vi "Version_4.9_8_on-chip_valves_for25ulSyringe_withModfied_Plunging.vi"() -> ()   [LabVIEW 2020] (continued)
                                tunnel: [w4564 w4571] -> w4555
                                tunnel: w4557 -> [w4563 w4572]
                                frame "Standard Pumping", Default {
                                n4147 = Subtract(x=w4565, y=w4566) -> (x-y=w4562:dbl)
                                n4148 = Absolute Value(x=w4562) -> (abs(x)=w4561:dbl)
                                n4149 = Multiply(x=w4561, y=w4563) -> (x*y=w4568:dbl)
                                n4150 = Divide(x=w4568, y=3000.0) -> (x/y=w4564:dbl)
                                }
                                frame "High Resolution Pumping" {
                                n4151 = Subtract(x=w4574, y=w4573) -> (x-y=w4570:dbl)
                                n4152 = Absolute Value(x=w4570) -> (abs(x)=w4569:dbl)
                                n4153 = Multiply(x=w4569, y=w4572) -> (x*y=w4576:dbl)
                                n4154 = Divide(x=w4576, y=24000.0) -> (x/y=w4571:dbl)
                                }
                                }
                                n4155 = local write "Volume being Injected \nin this process"(w4555) -> ()
                                }
                                frame #1 {
                                n4156 = call "LSPOneStatus (SubVI).vi"("VISA Refnum in"=w4580) -> ("read buffer"=w4582:string)  [unwired: 10 in]
                                n4157 = call <vilib>:"Trim Whitespace.vi"("string"=w4582) -> ("trimmed string"=w4581:string)  [unwired: 1 in]
                                n4158 = local read "Stopper that ends \nthe main loops"() -> (w4577:bool)
                                n4159 = Equal?(x=w4581, y="/0`\u0003") -> (x = y?=w4579:bool)
                                n4160 = Or(x=w4579, y=w4577) -> (x .or. y?=w4578:bool)
                                }
                                }
                                n4161 = Wait (ms)(milliseconds to wait=u32 100) -> ()  [unwired: 1 out]
                                n4162 = local read "Stopper that ends \nthe main loops"() -> (w4547:bool)
                                n4163 = case shown="True" w4547 {
                                frame False {
                                }
                                frame True {
                                n4164 = local read "VISA Refnum in\nfor Pump"() -> (w4554:refnum<visa-resource-name>)
                                n4165 = call "HardStopCurrentProcess (SubVI).vi"("VISA Refnum in"=w4554) -> ()  [unwired: 11 in]
                                }
                                }
                                }
                              }
                              frame #7 {
                                # "Change the pump port to Buffer-A1 for equilibriation of column-1"
                                n4166 = local read "VISA Refnum in\nfor Pump"() -> (w4585:refnum<visa-resource-name>)
                                n4167 = local read "Port for \nA1-Equilibriation"() -> (w4584:string)
                                n4168 = local write "Pause Data Collection"(TRUE ("Pause Data Collection")) -> ()
                                n4169 = Wait (ms)(milliseconds to wait=u32 500) -> ()  [unwired: 1 out]
                                n4170 = call "PortChanger (SubVI).vi"("Port Number"=w4584, "VISA Refnum in"=w4585) -> ()  [unwired: 10 in]
                              }
                              frame #8 {
                                n4171 = local read "VISA Refnum in\nfor Pump"() -> (w4589:refnum<visa-resource-name>)
                                n4172 = local write "Volume being Injected \nin this process"(0.0 ("Volume being Injected \nin this process")) -> ()
                                n4173 = call "ProcessCompletionWaiter (SubVI).vi"("VISA Refnum in"=w4589) -> ()  [unwired: 11 in]
                                n4174 = local write "Start the Process"(FALSE ("Start the Process")) -> ()
                              }
                            }
                          }
                          frame #7 {
                            # "Clean the tubing with Buffer-A1"
                            n4175 = local read "N-A1"() -> (w4591:i32)
                            n4176 = for {
                              N: w4591 -> [_]
                              n4177 = stacked-sequence {
                                frame #0 {
                                n4178 = local read "VISA Refnum in\nfor Pump"() -> (w4594:refnum<visa-resource-name>)
                                n4179 = local read "Port for \nA1-Equilibriation"() -> (w4593:string)
                                n4180 = call "PortChanger (SubVI).vi"("Port Number"=w4593, "VISA Refnum in"=w4594) -> ()  [unwired: 10 in]
                                }
                                frame #1 {
                                n4181 = local read "VISA Refnum in\nfor Pump"() -> (w4595:refnum<visa-resource-name>)
                                n4182 = call "ProcessCompletionWaiter (SubVI).vi"("VISA Refnum in"=w4595) -> ()  [unwired: 11 in]
                                }
                                frame #2 {
                                n4183 = local read "VISA Refnum in\nfor Pump"() -> (w4600:refnum<visa-resource-name>)
                                n4184 = local read "Apparent Volume\nof Syringe"() -> (w4596:dbl)
                                n4185 = local read "Volume of Syringe"() -> (w4597:dbl)
                                n4186 = call "RPickUp(SubVI).vi"("Volume to be picked up"=w4596, "Volume of Syringe"=w4597, "Resolution of PickUP"=T2."Standard Pumping", "PickUp Flow Rate (ul/min)"=150.0, "VISA Refnum in"=w4600) -> ()  [unwired: 6 in, 1 out]
                                }
                                frame #3 {
                                n4187 = local read "Stopper that ends \nthe main loops"() -> (w4601:bool)
                                n4188 = local read "VISA Refnum in\nfor Pump"() -> (w4602:refnum<visa-resource-name>)
                                n4189 = case shown="True" w4601 {
                                frame False {
                                }
                                frame True {
                                n4190 = local read "VISA Refnum in\nfor Pump"() -> (w4603:refnum<visa-resource-name>)
                                n4191 = call "HardStopCurrentProcess (SubVI).vi"("VISA Refnum in"=w4603) -> ()  [unwired: 11 in]
                                }
                                }
                                n4192 = call "ProcessCompletionWaiter (SubVI).vi"("VISA Refnum in"=w4602) -> ()  [unwired: 11 in]
                                }
                                frame #4 {
                                n4193 = local read "VISA Refnum in\nfor Pump"() -> (w4605:refnum<visa-resource-name>)
                                n4194 = call "PortChanger (SubVI).vi"("Port Number"="1", "VISA Refnum in"=w4605) -> ()  [unwired: 10 in]
                                }
                                frame #5 {
                                n4195 = local read "Stopper that ends \nthe main loops"() -> (w4606:bool)
                                n4196 = local read "VISA Refnum in\nfor Pump"() -> (w4607:refnum<visa-resource-name>)
                                n4197 = case shown="True" w4606 {
                                frame False {
                                }
                                frame True {
                                n4198 = local read "VISA Refnum in\nfor Pump"() -> (w4608:refnum<visa-resource-name>)
                                n4199 = call "HardStopCurrentProcess (SubVI).vi"("VISA Refnum in"=w4608) -> ()  [unwired: 11 in]
                                }
                                }
                                n4200 = call "ProcessCompletionWaiter (SubVI).vi"("VISA Refnum in"=w4607) -> ()  [unwired: 11 in]
                                }
                                frame #6 {
                                n4201 = local read "VISA Refnum in\nfor Pump"() -> (w4613:refnum<visa-resource-name>)
                                n4202 = local read "Volume of Syringe"() -> (w4610:dbl)
                                n4203 = call "GoToAbsolutePosition(SubVI).vi"("Absolute Volume Position in Syringe (in ul)"=0.0 ("Volume to be picked up"), "Volume of Syringe"=w4610, "Resolution of Pumping"=T2."Standard Pumping" ("Resolution of PickUP"), "Flow Rate (ul/min)"=150.0 ("PickUp Flow Rate (ul/min)"), "VISA Refnum in"=w4613) -> ()  [unwired: 6 in, 1 out]
                                }
                                frame #7 {
                                n4204 = local read "Stopper that ends \nthe main loops"() -> (w4614:bool)
                                n4205 = local read "VISA Refnum in\nfor Pump"() -> (w4615:refnum<visa-resource-name>)
                                n4206 = case shown="True" w4614 {
                                frame False {
                                }
                                frame True {
                                n4207 = local read "VISA Refnum in\nfor Pump"() -> (w4616:refnum<visa-resource-name>)
                                n4208 = call "HardStopCurrentProcess (SubVI).vi"("VISA Refnum in"=w4616) -> ()  [unwired: 11 in]
                                }
                                }
                                n4209 = call "ProcessCompletionWaiter (SubVI).vi"("VISA Refnum in"=w4615) -> ()  [unwired: 11 in]
                                }
                              }
                              n4210 = local write "Pause Data Collection"(TRUE ("Pause Data Collection")) -> ()
                            }
                          }
                          frame #8 {
                            # "Switch to Port-4"
                            # "Port-4 of pump is connected to Buffer-A1"
                            n4211 = local read "Port for \nA1-Equilibriation"() -> (w4617:string)
                            n4212 = local read "VISA Refnum in\nfor Pump"() -> (w4618:refnum<visa-resource-name>)
                            n4213 = call "PortChanger (SubVI).vi"("Port Number"=w4617, "VISA Refnum in"=w4618) -> ()  [unwired: 10 in]
                          }
                          frame #9 {
                            n4214 = local read "VISA Refnum in\nfor Pump"() -> (w4619:refnum<visa-resource-name>)
                            n4215 = call "ProcessCompletionWaiter (SubVI).vi"("VISA Refnum in"=w4619) -> ()  [unwired: 11 in]
                          }
                          frame #10 {
                            # "External vale is temporarily connected to teh waste outlet in this code"
                            n4216 = local write "Valve V3 Open"(FALSE ("Valve V3 Open")) -> ()
                            n4217 = local write "Valve V4 Open"(FALSE ("Valve V4 Open")) -> ()
                            n4218 = local write "Valve V1 Open"(TRUE ("Valve V1 Open")) -> ()
                            n4219 = local write "Valve V2 Open"(TRUE ("Valve V2 Open")) -> ()
                            n4220 = local write "External Valve \nOpen"(TRUE ("External Valve \nOpen")) -> ()
                            n4221 = local write "Valve V8 Open"(FALSE ("Valve V8 Open")) -> ()
                            n4222 = local write "Valve V6 Open"(FALSE ("Valve V6 Open")) -> ()
                            n4223 = local write "Valve V5 Open"(FALSE ("Valve V5 Open")) -> ()
                            n4224 = local write "Valve V7 Open"(FALSE ("Valve V7 Open")) -> ()
                          }
                          frame #11 {
                            n4225 = local read "Buffer-A1 Volume \nto be  Pumped \nfor Equilibration\nof Column-1"() -> (w4632:dbl)
                            n4226 = local read "Apparent Volume\nof Syringe"() -> (w4629:dbl)
                            n4227 = Quotient & Remainder(x=w4632, y=w4629) -> (x-y*floor(x/y)=w4630:dbl, floor(x/y)=w4631:dbl)
                            n4228 = for {
                              N: w4631 -> [_]
                              n4229 = stacked-sequence {
                                frame #0 {
                                n4230 = local read "Buffer-A1 PickUp \nFlow Rate (ul/min)\nfor Equilibration \nof Column-1"() -> (w4635:dbl)
                                n4231 = local read "Buffer-A1 Pumping\nResolution \nfor Equilibration \nof Column-1"() -> (w4634:T2)
                                n4232 = local read "VISA Refnum in\nfor Pump"() -> (w4637:refnum<visa-resource-name>)
                                n4233 = local read "Apparent Volume\nof Syringe"() -> (w4633:dbl)
                                n4234 = local read "Volume of Syringe"() -> (w4636:dbl)
                                n4235 = call "RPickUp(SubVI).vi"("Volume to be picked up"=w4633, "Volume of Syringe"=w4636, "Resolution of PickUP"=w4634, "PickUp Flow Rate (ul/min)"=w4635, "VISA Refnum in"=w4637) -> ()  [unwired: 6 in, 1 out]
                                }
                                frame #1 {
                                n4236 = while {
                                stop <- w4638 stop-if-true
                                n4237 = local read "Stopper that ends \nthe main loops"() -> (w4639:bool)
                                n4238 = local read "VISA Refnum in\nfor Pump"() -> (w4640:refnum<visa-resource-name>)
                                n4239 = case shown="True" w4639 {
                                frame False {
                                }
                                frame True {
                                n4240 = local read "VISA Refnum in\nfor Pump"() -> (w4641:refnum<visa-resource-name>)
                                n4241 = call "HardStopCurrentProcess (SubVI).vi"("VISA Refnum in"=w4641) -> ()  [unwired: 11 in]
                                }
                                }
                                n4242 = call "ProcessCompletionWaiterWithOutPut (SubVI).vi"("VISA Refnum in"=w4640) -> ("Boolean"=w4638:bool)  [unwired: 10 in]
                                }
                                }
                                frame #2 {
                                # "Reads the initial Plunger Position for computing the volume dispensed"
                                n4243 = local read "VISA Refnum in\nfor Pump"() -> (w4643:refnum<visa-resource-name>)
                                n4244 = call "AbsolutePlungerPosition (SubVI).vi"("VISA Refnum in"=w4643) -> ("Plunger Position"=w4642:i32)  [unwired: 10 in]
                                n4245 = local write "Initial Plunger Position"(w4642) -> ()
                                }
                                frame #3 {
                                # "Switch to Port-2"
                                # "Port-2 of the pump is conncted to column-1 of chip"
                                n4246 = local read "VISA Refnum in\nfor Pump"() -> (w4645:refnum<visa-resource-name>)
                                n4247 = call "PortChanger (SubVI).vi"("Port Number"="2", "VISA Refnum in"=w4645) -> ()  [unwired: 10 in]
                                }
                                frame #4 {
                                n4248 = while {
                                stop <- w4646 stop-if-true
                                n4249 = local read "Stopper that ends \nthe main loops"() -> (w4647:bool)
                                n4250 = local read "VISA Refnum in\nfor Pump"() -> (w4648:refnum<visa-resource-name>)
                                n4251 = case shown="True" w4647 {
                                frame False {
                                }
                                frame True {
                                n4252 = local read "VISA Refnum in\nfor Pump"() -> (w4649:refnum<visa-resource-name>)
                                n4253 = call "HardStopCurrentProcess (SubVI).vi"("VISA Refnum in"=w4649) -> ()  [unwired: 11 in]
                                }
                                }
                                n4254 = call "ProcessCompletionWaiterWithOutPut (SubVI).vi"("VISA Refnum in"=w4648) -> ("Boolean"=w4646:bool)  [unwired: 10 in]
                                }
                                }
                                frame #5 {
                                n4255 = local read "Buffer-A1 Dispense\nFlow Rate (ul/min) \nfor Equilibration\nof Column-1"() -> (w4653:dbl)
                                n4256 = local read "Buffer-A1 Pumping\nResolution \nfor Equilibration \nof Column-1"() -> (w4652:T2)
                                n4257 = local read "VISA Refnum in\nfor Pump"() -> (w4655:refnum<visa-resource-name>)
                                n4258 = local write "Pause Data Collection"(FALSE ("Pause Data Collection")) -> ()
                                n4259 = local read "Volume of Syringe"() -> (w4654:dbl)
                                n4260 = call "GoToAbsolutePosition(SubVI).vi"("Absolute Volume Position in Syringe (in ul)"=0.0, "Volume of Syringe"=w4654, "Resolution of Pumping"=w4652, "Flow Rate (ul/min)"=w4653, "VISA Refnum in"=w4655) -> ()  [unwired: 6 in, 1 out]
                                }
                                frame #6 {
                                n4261 = local read "Buffer-A1 Pumping\nResolution \nfor Equilibration \nof Column-1"() -> (w4657:T2)
                                n4262 = local read "VISA Refnum in\nfor Pump"() -> (w4659:refnum<visa-resource-name>)
                                n4263 = local read "Initial Plunger Position"() -> (w4658:dbl)
                                n4264 = local read "Volume of Syringe"() -> (w4656:dbl)
                                n4265 = while {
                                tunnel: w4658 -> [w4666]
                                tunnel: w4659 -> [w4665]
                                tunnel: w4657 -> [w4664]
                                tunnel: w4656 -> [w4663]
                                stop <- w4661 stop-if-true
                                n4266 = stacked-sequence {
                                tunnel: w4666 -> [w4673 _]
                                tunnel: w4665 -> [w4672 w4693]
                                tunnel: w4664 -> [w4671 _]
                                tunnel: w4663 -> [w4670 _]
                                tunnel: [_ w4691] -> w4661
                                frame #0 {
                                n4267 = call "AbsolutePlungerPosition (SubVI).vi"("VISA Refnum in"=w4672) -> ("Plunger Position"=w4669:i32)  [unwired: 10 in]
                                n4268 = case shown="\"Standard Pumping\", Default" w4671 {
                                tunnel: w4673 -> [w4678 w4687]
                                tunnel: w4669 -> [w4679 w4686]
                                tunnel: [w4677 w4684] -> w4668
                                tunnel: w4670 -> [w4676 w4685]
                                frame "Standard Pumping", Default {
                                n4269 = Subtract(x=w4678, y=w4679) -> (x-y=w4675:dbl)
                                n4270 = Absolute Value(x=w4675) -> (abs(x)=w4674:dbl)
                                n4271 = Multiply(x=w4674, y=w4676) -> (x*y=w4681:dbl)
                                n4272 = Divide(x=w4681, y=3000.0) -> (x/y=w4677:dbl)
                                }
                                frame "High Resolution Pumping" {
                                n4273 = Subtract(x=w4687, y=w4686) -> (x-y=w4683:dbl)
                                n4274 = Absolute Value(x=w4683) -> (abs(x)=w4682:dbl)
                                n4275 = Multiply(x=w4682, y=w4685) -> (x*y=w4689:dbl)
                                n4276 = Divide(x=w4689, y=24000.0) -> (x/y=w4684:dbl)
                                }
                                }
                                n4277 = local write "Volume being Injected \nin this process"(w4668) -> ()
                                }
                                frame #1 {
                                n4278 = call "LSPOneStatus (SubVI).vi"("VISA Refnum in"=w4693) -> ("read buffer"=w4695:string)  [unwired: 10 in]
                                n4279 = call <vilib>:"Trim Whitespace.vi"("string"=w4695) -> ("trimmed string"=w4694:string)  [unwired: 1 in]
                                n4280 = local read "Stopper that ends \nthe main loops"() -> (w4690:bool)
                                n4281 = Equal?(x=w4694, y="/0`\u0003") -> (x = y?=w4692:bool)
                                n4282 = Or(x=w4692, y=w4690) -> (x .or. y?=w4691:bool)
                                }
                                }
                                n4283 = Wait (ms)(milliseconds to wait=u32 100) -> ()  [unwired: 1 out]
                                n4284 = local read "Stopper that ends \nthe main loops"() -> (w4660:bool)
                                n4285 = case shown="True" w4660 {
                                frame False {
                                }
                                frame True {
                                n4286 = local read "VISA Refnum in\nfor Pump"() -> (w4667:refnum<visa-resource-name>)
                                n4287 = call "HardStopCurrentProcess (SubVI).vi"("VISA Refnum in"=w4667) -> ()  [unwired: 11 in]
                                }
                                }
                                }
                                }
                                frame #7 {
                                # "Change the pump port back to Buffer-A1"
                                n4288 = local read "VISA Refnum in\nfor Pump"() -> (w4698:refnum<visa-resource-name>)
                                n4289 = local read "Port for \nA1-Equilibriation"() -> (w4697:string)
                                n4290 = local write "Pause Data Collection"(TRUE ("Pause Data Collection")) -> ()
                                n4291 = Wait (ms)(milliseconds to wait=u32 500) -> ()  [unwired: 1 out]
                                n4292 = call "PortChanger (SubVI).vi"("Port Number"=w4697, "VISA Refnum in"=w4698) -> ()  [unwired: 10 in]
                                }
                                frame #8 {
                                n4293 = local read "VISA Refnum in\nfor Pump"() -> (w4701:refnum<visa-resource-name>)
                                n4294 = local write "Volume being Injected \nin this process"(0.0 ("Volume being Injected \nin this process")) -> ()
                                n4295 = call "ProcessCompletionWaiter (SubVI).vi"("VISA Refnum in"=w4701) -> ()  [unwired: 11 in]
                                }
                              }
                            }
                            n4296 = local write "Reminder of the \nVolume to be \nPumped"(w4630) -> ()
                          }
                          frame #12 {
                            n4297 = stacked-sequence {
                              frame #0 {
                                n4298 = local read "Buffer-A1 PickUp \nFlow Rate (ul/min)\nfor Equilibration \nof Column-1"() -> (w4705:dbl)
                                n4299 = local read "Buffer-A1 Pumping\nResolution \nfor Equilibration \nof Column-1"() -> (w4704:T2)
                                n4300 = local read "VISA Refnum in\nfor Pump"() -> (w4707:refnum<visa-resource-name>)
                                n4301 = local read "Reminder of the \nVolume to be \nPumped"() -> (w4703:dbl)
                                n4302 = local read "Volume of Syringe"() -> (w4706:dbl)
                                n4303 = call "RPickUp(SubVI).vi"("Volume to be picked up"=w4703, "Volume of Syringe"=w4706, "Resolution of PickUP"=w4704, "PickUp Flow Rate (ul/min)"=w4705, "VISA Refnum in"=w4707) -> ()  [unwired: 6 in, 1 out]
                              }
                              frame #1 {
                                n4304 = while {
                                stop <- w4708 stop-if-true
                                n4305 = local read "Stopper that ends \nthe main loops"() -> (w4709:bool)
                                n4306 = local read "VISA Refnum in\nfor Pump"() -> (w4710:refnum<visa-resource-name>)
                                n4307 = case shown="True" w4709 {
                                frame False {
                                }
                                frame True {
                                n4308 = local read "VISA Refnum in\nfor Pump"() -> (w4711:refnum<visa-resource-name>)
                                n4309 = call "HardStopCurrentProcess (SubVI).vi"("VISA Refnum in"=w4711) -> ()  [unwired: 11 in]
                                }
                                }
                                n4310 = call "ProcessCompletionWaiterWithOutPut (SubVI).vi"("VISA Refnum in"=w4710) -> ("Boolean"=w4708:bool)  [unwired: 10 in]
                                }
                              }
                              frame #2 {
                                # "Reads the initial Plunger Position for computing the volume dispensed"
                                n4311 = local read "VISA Refnum in\nfor Pump"() -> (w4713:refnum<visa-resource-name>)
                                n4312 = call "AbsolutePlungerPosition (SubVI).vi"("VISA Refnum in"=w4713) -> ("Plunger Position"=w4712:i32)  [unwired: 10 in]
                                n4313 = local write "Initial Plunger Position"(w4712) -> ()
                              }
                              frame #3 {
                                # "Switch to Port-2"
                                # "Port-2 of the pump is conncted to column-1 of chip"
                                n4314 = local read "VISA Refnum in\nfor Pump"() -> (w4715:refnum<visa-resource-name>)
                                n4315 = call "PortChanger (SubVI).vi"("Port Number"="2", "VISA Refnum in"=w4715) -> ()  [unwired: 10 in]
                              }
                              frame #4 {
                                n4316 = while {
                                stop <- w4716 stop-if-true
                                n4317 = local read "Stopper that ends \nthe main loops"() -> (w4717:bool)
                                n4318 = local read "VISA Refnum in\nfor Pump"() -> (w4718:refnum<visa-resource-name>)
                                n4319 = case shown="True" w4717 {
                                frame False {
                                }
                                frame True {
                                n4320 = local read "VISA Refnum in\nfor Pump"() -> (w4719:refnum<visa-resource-name>)
                                n4321 = call "HardStopCurrentProcess (SubVI).vi"("VISA Refnum in"=w4719) -> ()  [unwired: 11 in]
                                }
                                }
                                n4322 = call "ProcessCompletionWaiterWithOutPut (SubVI).vi"("VISA Refnum in"=w4718) -> ("Boolean"=w4716:bool)  [unwired: 10 in]
                                }
                              }
                              frame #5 {
                                n4323 = local read "Buffer-A1 Pumping\nResolution \nfor Equilibration \nof Column-1"() -> (w4722:T2)
                                n4324 = local read "Buffer-A1 Dispense\nFlow Rate (ul/min) \nfor Equilibration\nof Column-1"() -> (w4723:dbl)
                                n4325 = local read "VISA Refnum in\nfor Pump"() -> (w4725:refnum<visa-resource-name>)
                                n4326 = local write "Pause Data Collection"(FALSE ("Pause Data Collection")) -> ()
                                n4327 = local read "Volume of Syringe"() -> (w4724:dbl)
                                n4328 = call "GoToAbsolutePosition(SubVI).vi"("Absolute Volume Position in Syringe (in ul)"=0.0 ("Volume to be Dispensed"), "Volume of Syringe"=w4724, "Resolution of Pumping"=w4722, "Flow Rate (ul/min)"=w4723, "VISA Refnum in"=w4725) -> ()  [unwired: 6 in, 1 out]
                              }
                              frame #6 {
                                n4329 = local read "Buffer-A1 Pumping\nResolution \nfor Equilibration \nof Column-1"() -> (w4727:T2)
                                n4330 = local read "VISA Refnum in\nfor Pump"() -> (w4729:refnum<visa-resource-name>)
                                n4331 = local read "Initial Plunger Position"() -> (w4728:dbl)
                                n4332 = local read "Volume of Syringe"() -> (w4726:dbl)
                                n4333 = while {
                                tunnel: w4728 -> [w4736]
                                tunnel: w4729 -> [w4735]
                                tunnel: w4727 -> [w4734]
                                tunnel: w4726 -> [w4733]
                                stop <- w4731 stop-if-true
                                n4334 = stacked-sequence {
                                tunnel: w4736 -> [w4743 _]
                                tunnel: w4735 -> [w4742 w4763]
                                tunnel: w4734 -> [w4741 _]
                                tunnel: w4733 -> [w4740 _]
                                tunnel: [_ w4761] -> w4731
                                frame #0 {
                                n4335 = call "AbsolutePlungerPosition (SubVI).vi"("VISA Refnum in"=w4742) -> ("Plunger Position"=w4739:i32)  [unwired: 10 in]
                                n4336 = case shown="\"Standard Pumping\", Default" w4741 {
                                tunnel: w4743 -> [w4748 w4757]
                                tunnel: w4739 -> [w4749 w4756]
                                tunnel: [w4747 w4754] -> w4738
                                tunnel: w4740 -> [w4746 w4755]
                                frame "Standard Pumping", Default {
                                n4337 = Subtract(x=w4748, y=w4749) -> (x-y=w4745:dbl)
                                n4338 = Absolute Value(x=w4745) -> (abs(x)=w4744:dbl)
                                n4339 = Multiply(x=w4744, y=w4746) -> (x*y=w4751:dbl)
                                n4340 = Divide(x=w4751, y=3000.0) -> (x/y=w4747:dbl)
                                }
                                frame "High Resolution Pumping" {
                                n4341 = Subtract(x=w4757, y=w4756) -> (x-y=w4753:dbl)
                                n4342 = Absolute Value(x=w4753) -> (abs(x)=w4752:dbl)
                                n4343 = Multiply(x=w4752, y=w4755) -> (x*y=w4759:dbl)
                                n4344 = Divide(x=w4759, y=24000.0) -> (x/y=w4754:dbl)
                                }
                                }
                                n4345 = local write "Volume being Injected \nin this process"(w4738) -> ()
                                }
                                frame #1 {
                                n4346 = call "LSPOneStatus (SubVI).vi"("VISA Refnum in"=w4763) -> ("read buffer"=w4765:string)  [unwired: 10 in]
                                n4347 = call <vilib>:"Trim Whitespace.vi"("string"=w4765) -> ("trimmed string"=w4764:string)  [unwired: 1 in]
                                n4348 = local read "Stopper that ends \nthe main loops"() -> (w4760:bool)
                                n4349 = Equal?(x=w4764, y="/0`\u0003") -> (x = y?=w4762:bool)
                                n4350 = Or(x=w4762, y=w4760) -> (x .or. y?=w4761:bool)
                                }
                                }
                                n4351 = Wait (ms)(milliseconds to wait=u32 100) -> ()  [unwired: 1 out]
                                n4352 = local read "Stopper that ends \nthe main loops"() -> (w4730:bool)
                                n4353 = case shown="True" w4730 {
                                frame False {
                                }
                                frame True {
                                n4354 = local read "VISA Refnum in\nfor Pump"() -> (w4737:refnum<visa-resource-name>)
                                n4355 = call "HardStopCurrentProcess (SubVI).vi"("VISA Refnum in"=w4737) -> ()  [unwired: 11 in]
                                }
                                }
                                }
                              }
                              frame #7 {
                                # "Change the pump port to Buffer-C1 for equilibriation of column-2"
                                n4356 = local read "VISA Refnum in\nfor Pump"() -> (w4768:refnum<visa-resource-name>)
                                n4357 = local read "Port for \nC1-Equilibriation"() -> (w4767:string)
                                n4358 = local write "Pause Data Collection"(TRUE ("Pause Data Collection")) -> ()
                                n4359 = Wait (ms)(milliseconds to wait=u32 500) -> ()  [unwired: 1 out]
                                n4360 = call "PortChanger (SubVI).vi"("Port Number"=w4767, "VISA Refnum in"=w4768) -> ()  [unwired: 10 in]
                              }
                              frame #8 {
                                n4361 = local read "VISA Refnum in\nfor Pump"() -> (w4772:refnum<visa-resource-name>)
                                n4362 = local write "Volume being Injected \nin this process"(0.0 ("Volume being Injected \nin this process")) -> ()
                                n4363 = call "ProcessCompletionWaiter (SubVI).vi"("VISA Refnum in"=w4772) -> ()  [unwired: 11 in]
                                n4364 = local write "Start the Process"(FALSE ("Start the Process")) -> ()
                              }
                            }
                          }
                          frame #13 {
                            # "Clean the tubing with Buffer-C1"
                            n4365 = local read "N-C1"() -> (w4775:i32)
                            n4366 = local write "Equilibriating \nColumn-1"(FALSE ("Equilibriating \nColumn-1")) -> ()
                            n4367 = for {
                              N: w4775 -> [_]
                              n4368 = stacked-sequence {
                                frame #0 {
                                n4369 = local read "Port for \nC1-Equilibriation"() -> (w4778:string)
                                n4370 = local read "VISA Refnum in\nfor Pump"() -> (w4779:refnum<visa-resource-name>)
                                n4371 = call "PortChanger (SubVI).vi"("Port Number"=w4778, "VISA Refnum in"=w4779) -> ()  [unwired: 10 in]
                                }
                                frame #1 {
                                n4372 = local read "VISA Refnum in\nfor Pump"() -> (w4780:refnum<visa-resource-name>)
                                n4373 = call "ProcessCompletionWaiter (SubVI).vi"("VISA Refnum in"=w4780) -> ()  [unwired: 11 in]
                                }
                                frame #2 {
                                n4374 = local read "VISA Refnum in\nfor Pump"() -> (w4785:refnum<visa-resource-name>)
                                n4375 = local read "Apparent Volume\nof Syringe"() -> (w4781:dbl)
                                n4376 = local read "Volume of Syringe"() -> (w4782:dbl)
                                n4377 = call "RPickUp(SubVI).vi"("Volume to be picked up"=w4781, "Volume of Syringe"=w4782, "Resolution of PickUP"=T2."Standard Pumping", "PickUp Flow Rate (ul/min)"=150.0, "VISA Refnum in"=w4785) -> ()  [unwired: 6 in, 1 out]
                                }
                                frame #3 {
                                n4378 = local read "Stopper that ends \nthe main loops"() -> (w4786:bool)
                                n4379 = local read "VISA Refnum in\nfor Pump"() -> (w4787:refnum<visa-resource-name>)
                                n4380 = case shown="True" w4786 {
                                frame False {
                                }
                                frame True {
                                n4381 = local read "VISA Refnum in\nfor Pump"() -> (w4788:refnum<visa-resource-name>)
                                n4382 = call "HardStopCurrentProcess (SubVI).vi"("VISA Refnum in"=w4788) -> ()  [unwired: 11 in]
                                }
                                }
                                n4383 = call "ProcessCompletionWaiter (SubVI).vi"("VISA Refnum in"=w4787) -> ()  [unwired: 11 in]
                                }
                                frame #4 {
                                n4384 = local read "VISA Refnum in\nfor Pump"() -> (w4790:refnum<visa-resource-name>)
                                n4385 = call "PortChanger (SubVI).vi"("Port Number"="1", "VISA Refnum in"=w4790) -> ()  [unwired: 10 in]
                                }
                                frame #5 {
                                n4386 = local read "Stopper that ends \nthe main loops"() -> (w4791:bool)
                                n4387 = local read "VISA Refnum in\nfor Pump"() -> (w4792:refnum<visa-resource-name>)
                                n4388 = case shown="True" w4791 {
                                frame False {
                                }
                                frame True {
                                n4389 = local read "VISA Refnum in\nfor Pump"() -> (w4793:refnum<visa-resource-name>)
                                n4390 = call "HardStopCurrentProcess (SubVI).vi"("VISA Refnum in"=w4793) -> ()  [unwired: 11 in]
                                }
                                }
                                n4391 = call "ProcessCompletionWaiter (SubVI).vi"("VISA Refnum in"=w4792) -> ()  [unwired: 11 in]
                                }
                                frame #6 {
                                n4392 = local read "VISA Refnum in\nfor Pump"() -> (w4798:refnum<visa-resource-name>)
                                n4393 = local read "Volume of Syringe"() -> (w4795:dbl)
                                n4394 = call "GoToAbsolutePosition(SubVI).vi"("Absolute Volume Position in Syringe (in ul)"=0.0 ("Volume to be picked up"), "Volume of Syringe"=w4795, "Resolution of Pumping"=T2."Standard Pumping" ("Resolution of PickUP"), "Flow Rate (ul/min)"=150.0 ("PickUp Flow Rate (ul/min)"), "VISA Refnum in"=w4798) -> ()  [unwired: 6 in, 1 out]
                                }
                                frame #7 {
                                n4395 = local read "Stopper that ends \nthe main loops"() -> (w4799:bool)
                                n4396 = local read "VISA Refnum in\nfor Pump"() -> (w4800:refnum<visa-resource-name>)
                                n4397 = case shown="True" w4799 {
                                frame False {
                                }
                                frame True {
                                n4398 = local read "VISA Refnum in\nfor Pump"() -> (w4801:refnum<visa-resource-name>)
                                n4399 = call "HardStopCurrentProcess (SubVI).vi"("VISA Refnum in"=w4801) -> ()  [unwired: 11 in]
                                }
                                }
                                n4400 = call "ProcessCompletionWaiter (SubVI).vi"("VISA Refnum in"=w4800) -> ()  [unwired: 11 in]
                                }
                              }
                            }
                            n4401 = local write "Pause Data Collection"(TRUE ("Pause Data Collection")) -> ()
                            n4402 = local write "Equilibriating \nColumn-2"(TRUE ("Equilibriating \nColumn-2")) -> ()
                          }
                          frame #14 {
                            n4403 = local read "Buffer-C1 Volume \nto be  Pumped \nfor Equilibration\nof Column-2"() -> (w4805:dbl)
                            n4404 = local read "Apparent Volume\nof Syringe"() -> (w4802:dbl)
                            n4405 = Quotient & Remainder(x=w4805, y=w4802) -> (x-y*floor(x/y)=w4803:dbl, floor(x/y)=w4804:dbl)
                            n4406 = for {
                              N: w4804 -> [_]
                              n4407 = stacked-sequence {
                                frame #0 {
                                n4408 = local read "VISA Refnum in\nfor Pump"() -> (w4807:refnum<visa-resource-name>)
                                n4409 = local read "Port for \nC1-Equilibriation"() -> (w4806:string)
                                n4410 = call "PortChanger (SubVI).vi"("Port Number"=w4806, "VISA Refnum in"=w4807) -> ()  [unwired: 10 in]
                                }
                                frame #1 {
                                n4411 = local read "VISA Refnum in\nfor Pump"() -> (w4808:refnum<visa-resource-name>)
                                n4412 = call "ProcessCompletionWaiter (SubVI).vi"("VISA Refnum in"=w4808) -> ()  [unwired: 11 in]
                                }
                                frame #2 {
                                n4413 = local read "Buffer-C1 PickUp \nFlow Rate (ul/min)\nfor Equilibration \nof Column-2"() -> (w4811:dbl)
                                n4414 = local read "Buffer-C1 Pumping\nResolution \nfor Equilibration \nof Column-2"() -> (w4810:T2)
                                n4415 = local read "VISA Refnum in\nfor Pump"() -> (w4813:refnum<visa-resource-name>)
                                n4416 = local read "Apparent Volume\nof Syringe"() -> (w4809:dbl)
                                n4417 = local read "Volume of Syringe"() -> (w4812:dbl)
                                n4418 = call "RPickUp(SubVI).vi"("Volume to be picked up"=w4809, "Volume of Syringe"=w4812, "Resolution of PickUP"=w4810, "PickUp Flow Rate (ul/min)"=w4811, "VISA Refnum in"=w4813) -> ()  [unwired: 6 in, 1 out]
                                }
                                frame #3 {
                                n4419 = while {
                                stop <- w4814 stop-if-true
                                n4420 = local read "Stopper that ends \nthe main loops"() -> (w4815:bool)
                                n4421 = local read "VISA Refnum in\nfor Pump"() -> (w4816:refnum<visa-resource-name>)
                                n4422 = case shown="True" w4815 {
                                frame False {
                                }
                                frame True {
                                n4423 = local read "VISA Refnum in\nfor Pump"() -> (w4817:refnum<visa-resource-name>)
                                n4424 = call "HardStopCurrentProcess (SubVI).vi"("VISA Refnum in"=w4817) -> ()  [unwired: 11 in]
                                }
                                }
                                n4425 = call "ProcessCompletionWaiterWithOutPut (SubVI).vi"("VISA Refnum in"=w4816) -> ("Boolean"=w4814:bool)  [unwired: 10 in]
                                }
                                }
                                frame #4 {
                                # "Reads the initial Plunger Position for computing the volume dispensed"
                                n4426 = local read "VISA Refnum in\nfor Pump"() -> (w4819:refnum<visa-resource-name>)
                                n4427 = call "AbsolutePlungerPosition (SubVI).vi"("VISA Refnum in"=w4819) -> ("Plunger Position"=w4818:i32)  [unwired: 10 in]
                                n4428 = local write "Initial Plunger Position"(w4818) -> ()
                                }
                                frame #5 {
                                # "Switch to Port-10"
                                # "Port-10 of the pump is conncted to column-2 of chip"
                                n4429 = local read "VISA Refnum in\nfor Pump"() -> (w4821:refnum<visa-resource-name>)
                                n4430 = call "PortChanger (SubVI).vi"("Port Number"="10", "VISA Refnum in"=w4821) -> ()  [unwired: 10 in]
                                }
                                frame #6 {
                                n4431 = while {
                                stop <- w4822 stop-if-true
                                n4432 = local read "Stopper that ends \nthe main loops"() -> (w4823:bool)
                                n4433 = local read "VISA Refnum in\nfor Pump"() -> (w4824:refnum<visa-resource-name>)
                                n4434 = case shown="True" w4823 {
                                frame False {
                                }
                                frame True {
                                n4435 = local read "VISA Refnum in\nfor Pump"() -> (w4825:refnum<visa-resource-name>)
                                n4436 = call "HardStopCurrentProcess (SubVI).vi"("VISA Refnum in"=w4825) -> ()  [unwired: 11 in]
                                }
                                }
                                n4437 = call "ProcessCompletionWaiterWithOutPut (SubVI).vi"("VISA Refnum in"=w4824) -> ("Boolean"=w4822:bool)  [unwired: 10 in]
                                }
                                }
                                frame #7 {
                                # "Buffer-C pumped for column non-interference"
                                # "Keeps the AMF valve after column-1 open and valve after column-2 closed"
                                n4438 = local read "Buffer-C1 Dispense\nFlow Rate (ul/min) \nfor Equilibration\nof Column-2"() -> (w4838:dbl)
                                n4439 = local read "Buffer-C1 Pumping\nResolution \nfor Equilibration \nof Column-2"() -> (w4837:T2)
                                n4440 = local read "VISA Refnum in\nfor Pump"() -> (w4840:refnum<visa-resource-name>)
                                n4441 = local write "Pause Data Collection"(FALSE ("Pause Data Collection")) -> ()
                                n4442 = local read "Volume of Syringe"() -> (w4839:dbl)
                                n4443 = call "GoToAbsolutePosition(SubVI).vi"("Absolute Volume Position in Syringe (in ul)"=0.0, "Volume of Syringe"=w4839, "Resolution of Pumping"=w4837, "Flow Rate (ul/min)"=w4838, "VISA Refnum in"=w4840) -> ()  [unwired: 6 in, 1 out]
                                n4444 = local write "Valve V1 Open"(FALSE ("Valve V1 Open")) -> ()
                                n4445 = local write "Valve V2 Open"(TRUE ("Valve V2 Open")) -> ()
                                n4446 = local write "Valve V4 Open"(FALSE ("Valve V4 Open")) -> ()
                                n4447 = local write "Valve V3 Open"(TRUE ("Valve V3 Open")) -> ()
                                n4448 = local write "External Valve \nOpen"(TRUE ("External Valve \nOpen")) -> ()
                                n4449 = local write "Valve V5 Open"(FALSE ("Valve V5 Open")) -> ()
                                n4450 = local write "Valve V6 Open"(FALSE ("Valve V6 Open")) -> ()
                                n4451 = local write "Valve V7 Open"(FALSE ("Valve V7 Open")) -> ()
                                n4452 = local write "Valve V8 Open"(FALSE ("Valve V8 Open")) -> ()
                                }
                                frame #8 {
                                n4453 = local read "Buffer-C1 Pumping\nResolution \nfor Equilibration \nof Column-2"() -> (w4842:T2)
                                n4454 = local read "VISA Refnum in\nfor Pump"() -> (w4844:refnum<visa-resource-name>)
                                n4455 = local read "Initial Plunger Position"() -> (w4843:dbl)
                                n4456 = local read "Volume of Syringe"() -> (w4841:dbl)
                                n4457 = while {
                                tunnel: w4843 -> [w4851]
                                tunnel: w4844 -> [w4850]
                                tunnel: w4842 -> [w4849]
                                tunnel: w4841 -> [w4848]
                                stop <- w4846 stop-if-true
                                n4458 = stacked-sequence {
                                tunnel: w4851 -> [w4858 _]
                                tunnel: w4850 -> [w4857 w4882]
                                tunnel: w4849 -> [w4856 _]
                                tunnel: w4848 -> [w4855 _]
                                tunnel: [_ w4880] -> w4846
                                frame #0 {
                                n4459 = call "AbsolutePlungerPosition (SubVI).vi"("VISA Refnum in"=w4857) -> ("Plunger Position"=w4854:i32)  [unwired: 10 in]
                                n4460 = case shown="\"Standard Pumping\", Default" w4856 {
                                tunnel: w4858 -> [w4863 w4872]
                                tunnel: w4854 -> [w4864 w4871]
                                tunnel: [w4862 w4869] -> w4853
                                tunnel: w4855 -> [w4861 w4870]
                                frame "Standard Pumping", Default {
                                n4461 = Subtract(x=w4863, y=w4864) -> (x-y=w4860:dbl)
                                n4462 = Absolute Value(x=w4860) -> (abs(x)=w4859:dbl)
                                n4463 = Multiply(x=w4859, y=w4861) -> (x*y=w4866:dbl)
                                n4464 = Divide(x=w4866, y=3000.0) -> (x/y=w4862:dbl)
                                }
                                frame "High Resolution Pumping" {
                                n4465 = Subtract(x=w4872, y=w4871) -> (x-y=w4868:dbl)
                                n4466 = Absolute Value(x=w4868) -> (abs(x)=w4867:dbl)
                                n4467 = Multiply(x=w4867, y=w4870) -> (x*y=w4874:dbl)
                                n4468 = Divide(x=w4874, y=24000.0) -> (x/y=w4869:dbl)
                                }
                                }
                                n4469 = local write "Volume being Injected \nin this process"(w4853) -> ()
                                }
                                frame #1 {
                                n4470 = local read "Buffer-C Volume \nto be Pumped for\nColumn \nnon-interference"() -> (w4878:dbl)
                                n4471 = local read "Volume being Injected \nin this process"() -> (w4879:dbl)
                                n4472 = local read "Stopper that ends \nthe main loops"() -> (w4877:bool)
                                n4473 = call "LSPOneStatus (SubVI).vi"("VISA Refnum in"=w4882) -> ("read buffer"=w4884:string)  [unwired: 10 in]
                                n4474 = call <vilib>:"Trim Whitespace.vi"("string"=w4884) -> ("trimmed string"=w4883:string)  [unwired: 1 in]
                                n4475 = Equal?(x=w4883, y="/0`\u0003") -> (x = y?=w4881:bool)
                                n4476 = Greater Or Equal?(x=w4879, y=w4878) -> (x >= y?=w4876:bool)
                                n4477 = Or(x=w4877, y=w4876) -> (x .or. y?=w4875:bool)
                                n4478 = Or(x=w4881, y=w4875) -> (x .or. y?=w4880:bool)
                                }
                                }
                                n4479 = Wait (ms)(milliseconds to wait=u32 100) -> ()  [unwired: 1 out]
                                n4480 = local read "Stopper that ends \nthe main loops"() -> (w4845:bool)
                                n4481 = case shown="True" w4845 {
                                frame False {
                                }
                                frame True {
                                n4482 = local read "VISA Refnum in\nfor Pump"() -> (w4852:refnum<visa-resource-name>)
                                n4483 = call "HardStopCurrentProcess (SubVI).vi"("VISA Refnum in"=w4852) -> ()  [unwired: 11 in]
                                }
                                }
                                }
                                }
                                frame #9 {
                                n4484 = local write "Valve V3 Open"(TRUE ("Valve V3 Open")) -> ()
                                n4485 = local write "Valve V2 Open"(FALSE ("Valve V2 Open")) -> ()
                                n4486 = local write "Valve V4 Open"(TRUE ("Valve V1 Open")) -> ()
                                n4487 = local write "Valve V1 Open"(FALSE ("Valve V1 Open")) -> ()
                                n4488 = local write "External Valve \nOpen"(FALSE ("External Valve \nOpen")) -> ()
                                n4489 = local write "Valve V5 Open"(TRUE ("Valve V4 Open")) -> ()
                                n4490 = local write "Valve V8 Open"(FALSE ("Valve V8 Open")) -> ()
                                n4491 = local write "Valve V7 Open"(TRUE ("Valve V6 Open")) -> ()
                                n4492 = local write "Valve V6 Open"(FALSE ("Valve V6 Open")) -> ()
                                }
                                frame #10 {
                                n4493 = local read "Buffer-C1 Pumping\nResolution \nfor Equilibration \nof Column-2"() -> (w4896:T2)
                                n4494 = local read "VISA Refnum in\nfor Pump"() -> (w4898:refnum<visa-resource-name>)
                                n4495 = local read "Initial Plunger Position"() -> (w4897:dbl)
                                n4496 = local read "Volume of Syringe"() -> (w4895:dbl)
                                n4497 = while {
                                tunnel: w4897 -> [w4905]
                                tunnel: w4898 -> [w4904]
                                tunnel: w4896 -> [w4903]
                                tunnel: w4895 -> [w4902]
                                stop <- w4900 stop-if-true
                                n4498 = stacked-sequence {
                                tunnel: w4905 -> [w4912 _]
                                tunnel: w4904 -> [w4911 w4932]
                                tunnel: w4903 -> [w4910 _]
                                tunnel: w4902 -> [w4909 _]
                                tunnel: [_ w4930] -> w4900
                                frame #0 {
                                n4499 = call "AbsolutePlungerPosition (SubVI).vi"("VISA Refnum in"=w4911) -> ("Plunger Position"=w4908:i32)  [unwired: 10 in]
                                n4500 = case shown="\"Standard Pumping\", Default" w4910 {
                                tunnel: w4912 -> [w4917 w4926]
                                tunnel: w4908 -> [w4918 w4925]
                                tunnel: [w4916 w4923] -> w4907
                                tunnel: w4909 -> [w4915 w4924]
                                frame "Standard Pumping", Default {
                                n4501 = Subtract(x=w4917, y=w4918) -> (x-y=w4914:dbl)
                                n4502 = Absolute Value(x=w4914) -> (abs(x)=w4913:dbl)
                                n4503 = Multiply(x=w4913, y=w4915) -> (x*y=w4920:dbl)
                                n4504 = Divide(x=w4920, y=3000.0) -> (x/y=w4916:dbl)
                                }
                                frame "High Resolution Pumping" {
                                n4505 = Subtract(x=w4926, y=w4925) -> (x-y=w4922:dbl)
                                n4506 = Absolute Value(x=w4922) -> (abs(x)=w4921:dbl)
                                n4507 = Multiply(x=w4921, y=w4924) -> (x*y=w4928:dbl)
                                n4508 = Divide(x=w4928, y=24000.0) -> (x/y=w4923:dbl)
                                }
                                }
                                n4509 = local write "Volume being Injected \nin this process"(w4907) -> ()
                                }
                                frame #1 {
                                n4510 = local read "Stopper that ends \nthe main loops"() -> (w4929:bool)
                                n4511 = call "LSPOneStatus (SubVI).vi"("VISA Refnum in"=w4932) -> ("read buffer"=w4934:string)  [unwired: 10 in]
                                n4512 = call <vilib>:"Trim Whitespace.vi"("string"=w4934) -> ("trimmed string"=w4933:string)  [unwired: 1 in]
                                n4513 = Equal?(x=w4933, y="/0`\u0003") -> (x = y?=w4931:bool)
                                n4514 = Or(x=w4931, y=w4929) -> (x .or. y?=w4930:bool)
                                }
                                }
                                n4515 = Wait (ms)(milliseconds to wait=u32 100) -> ()  [unwired: 1 out]
                                n4516 = local read "Stopper that ends \nthe main loops"() -> (w4899:bool)
                                n4517 = case shown="True" w4899 {
                                frame False {
                                }
                                frame True {
                                n4518 = local read "VISA Refnum in\nfor Pump"() -> (w4906:refnum<visa-resource-name>)
                                n4519 = call "HardStopCurrentProcess (SubVI).vi"("VISA Refnum in"=w4906) -> ()  [unwired: 11 in]
                                }
                                }
                                }
                                }
                                frame #11 {
                                # "Change the pump port back to Buffer-C1"
                                n4520 = local read "VISA Refnum in\nfor Pump"() -> (w4937:refnum<visa-resource-name>)
                                n4521 = local read "Port for \nC1-Equilibriation"() -> (w4936:string)
                                n4522 = local write "Pause Data Collection"(TRUE ("Pause Data Collection")) -> ()
                                n4523 = Wait (ms)(milliseconds to wait=u32 500) -> ()  [unwired: 1 out]
                                n4524 = call "PortChanger (SubVI).vi"("Port Number"=w4936, "VISA Refnum in"=w4937) -> ()  [unwired: 10 in]
                                }
                                frame #12 {
                                n4525 = local read "VISA Refnum in\nfor Pump"() -> (w4940:refnum<visa-resource-name>)
                                n4526 = local write "Volume being Injected \nin this process"(0.0 ("Volume being Injected \nin this process")) -> ()
                                n4527 = call "ProcessCompletionWaiter (SubVI).vi"("VISA Refnum in"=w4940) -> ()  [unwired: 11 in]
                                }
                              }
                            }
                            n4528 = local write "Reminder of the \nVolume to be \nPumped"(w4803) -> ()
                          }
                          frame #15 {
                            n4529 = stacked-sequence {
                              frame #0 {
                                n4530 = local read "Buffer-C1 PickUp \nFlow Rate (ul/min)\nfor Equilibration \nof Column-2"() -> (w4944:dbl)
                                n4531 = local read "Buffer-C1 Pumping\nResolution \nfor Equilibration \nof Column-2"() -> (w4943:T2)
                                n4532 = local read "VISA Refnum in\nfor Pump"() -> (w4946:refnum<visa-resource-name>)
                                n4533 = local read "Reminder of the \nVolume to be \nPumped"() -> (w4942:dbl)
                                n4534 = local read "Volume of Syringe"() -> (w4945:dbl)
                                n4535 = call "RPickUp(SubVI).vi"("Volume to be picked up"=w4942, "Volume of Syringe"=w4945, "Resolution of PickUP"=w4943, "PickUp Flow Rate (ul/min)"=w4944, "VISA Refnum in"=w4946) -> ()  [unwired: 6 in, 1 out]
                              }
                              frame #1 {
                                n4536 = while {
                                stop <- w4947 stop-if-true
                                n4537 = local read "Stopper that ends \nthe main loops"() -> (w4948:bool)
                                n4538 = local read "VISA Refnum in\nfor Pump"() -> (w4949:refnum<visa-resource-name>)
                                n4539 = case shown="True" w4948 {
                                frame False {
                                }
                                frame True {
                                n4540 = local read "VISA Refnum in\nfor Pump"() -> (w4950:refnum<visa-resource-name>)
                                n4541 = call "HardStopCurrentProcess (SubVI).vi"("VISA Refnum in"=w4950) -> ()  [unwired: 11 in]
                                }
                                }
                                n4542 = call "ProcessCompletionWaiterWithOutPut (SubVI).vi"("VISA Refnum in"=w4949) -> ("Boolean"=w4947:bool)  [unwired: 10 in]
                                }
                              }
                              frame #2 {
                                # "Reads the initial Plunger Position for computing the volume dispensed"
                                n4543 = local read "VISA Refnum in\nfor Pump"() -> (w4952:refnum<visa-resource-name>)
                                n4544 = call "AbsolutePlungerPosition (SubVI).vi"("VISA Refnum in"=w4952) -> ("Plunger Position"=w4951:i32)  [unwired: 10 in]
                                n4545 = local write "Initial Plunger Position"(w4951) -> ()
                              }
                              frame #3 {
                                # "Switch to Port-10"
                                # "Port-10 of the pump is conncted to column-2 of chip"
                                n4546 = local read "VISA Refnum in\nfor Pump"() -> (w4954:refnum<visa-resource-name>)
                                n4547 = call "PortChanger (SubVI).vi"("Port Number"="10", "VISA Refnum in"=w4954) -> ()  [unwired: 10 in]
                              }
                              frame #4 {
                                n4548 = while {
                                stop <- w4955 stop-if-true
                                n4549 = local read "Stopper that ends \nthe main loops"() -> (w4956:bool)
                                n4550 = local read "VISA Refnum in\nfor Pump"() -> (w4957:refnum<visa-resource-name>)
                                n4551 = case shown="True" w4956 {
                                frame False {
                                }
                                frame True {
                                n4552 = local read "VISA Refnum in\nfor Pump"() -> (w4958:refnum<visa-resource-name>)
                                n4553 = call "HardStopCurrentProcess (SubVI).vi"("VISA Refnum in"=w4958) -> ()  [unwired: 11 in]
                                }
                                }
                                n4554 = call "ProcessCompletionWaiterWithOutPut (SubVI).vi"("VISA Refnum in"=w4957) -> ("Boolean"=w4955:bool)  [unwired: 10 in]
                                }
                              }
                              frame #5 {
                                # "Keeps the AMF valve after column-1 open and valve after column-2 closed"
                                n4555 = local read "Buffer-C1 Dispense\nFlow Rate (ul/min) \nfor Equilibration\nof Column-2"() -> (w4971:dbl)
                                n4556 = local read "Buffer-C1 Pumping\nResolution \nfor Equilibration \nof Column-2"() -> (w4970:T2)
                                n4557 = local read "VISA Refnum in\nfor Pump"() -> (w4973:refnum<visa-resource-name>)
                                n4558 = local write "Pause Data Collection"(FALSE ("Pause Data Collection")) -> ()
                                n4559 = local read "Volume of Syringe"() -> (w4972:dbl)
                                n4560 = call "GoToAbsolutePosition(SubVI).vi"("Absolute Volume Position in Syringe (in ul)"=0.0, "Volume of Syringe"=w4972, "Resolution of Pumping"=w4970, "Flow Rate (ul/min)"=w4971, "VISA Refnum in"=w4973) -> ()  [unwired: 6 in, 1 out]
                                n4561 = local write "Valve V1 Open"(FALSE ("Valve V1 Open")) -> ()
                                n4562 = local write "Valve V2 Open"(TRUE ("Valve V2 Open")) -> ()
                                n4563 = local write "Valve V3 Open"(TRUE ("Valve V3 Open")) -> ()
                                n4564 = local write "Valve V4 Open"(FALSE ("Affinity On")) -> ()
                                n4565 = local write "External Valve \nOpen"(TRUE ("External Valve \nOpen")) -> ()
                                n4566 = local write "Valve V8 Open"(FALSE ("Valve V8 Open")) -> ()
                                n4567 = local write "Valve V5 Open"(FALSE ("Valve V5 Open")) -> ()
                                n4568 = local write "Valve V6 Open"(FALSE ("Valve V6 Open")) -> ()
                                n4569 = local write "Valve V7 Open"(FALSE ("Valve V7 Open")) -> ()
                              }
                              frame #6 {
                                n4570 = local read "Buffer-C1 Pumping\nResolution \nfor Equilibration \nof Column-2"() -> (w4975:T2)
                                n4571 = local read "VISA Refnum in\nfor Pump"() -> (w4977:refnum<visa-resource-name>)
                                n4572 = local read "Initial Plunger Position"() -> (w4976:dbl)
                                n4573 = local read "Volume of Syringe"() -> (w4974:dbl)
                                n4574 = while {
                                tunnel: w4976 -> [w4984]
                                tunnel: w4977 -> [w4983]
                                tunnel: w4975 -> [w4982]
                                tunnel: w4974 -> [w4981]
                                stop <- w4979 stop-if-true
                                n4575 = stacked-sequence {
                                tunnel: w4984 -> [w4991 _]
                                tunnel: w4983 -> [w4990 w5015]
                                tunnel: w4982 -> [w4989 _]
                                tunnel: w4981 -> [w4988 _]
                                tunnel: [_ w5013] -> w4979
                                frame #0 {
                                n4576 = call "AbsolutePlungerPosition (SubVI).vi"("VISA Refnum in"=w4990) -> ("Plunger Position"=w4987:i32)  [unwired: 10 in]
                                n4577 = case shown="\"Standard Pumping\", Default" w4989 {
                                tunnel: w4991 -> [w4996 w5005]
                                tunnel: w4987 -> [w4997 w5004]
                                tunnel: [w4995 w5002] -> w4986
                                tunnel: w4988 -> [w4994 w5003]
                                frame "Standard Pumping", Default {
                                n4578 = Subtract(x=w4996, y=w4997) -> (x-y=w4993:dbl)
                                n4579 = Absolute Value(x=w4993) -> (abs(x)=w4992:dbl)
                                n4580 = Multiply(x=w4992, y=w4994) -> (x*y=w4999:dbl)
                                n4581 = Divide(x=w4999, y=3000.0) -> (x/y=w4995:dbl)
                                }
                                frame "High Resolution Pumping" {
                                n4582 = Subtract(x=w5005, y=w5004) -> (x-y=w5001:dbl)
                                n4583 = Absolute Value(x=w5001) -> (abs(x)=w5000:dbl)
                                n4584 = Multiply(x=w5000, y=w5003) -> (x*y=w5007:dbl)
                                n4585 = Divide(x=w5007, y=24000.0) -> (x/y=w5002:dbl)
                                }
                                }
                                n4586 = local write "Volume being Injected \nin this process"(w4986) -> ()
                                }
                                frame #1 {
                                n4587 = local read "Buffer-C Volume \nto be Pumped for\nColumn \nnon-interference"() -> (w5011:dbl)
                                n4588 = local read "Volume being Injected \nin this process"() -> (w5012:dbl)
                                n4589 = local read "Stopper that ends \nthe main loops"() -> (w5010:bool)
                                n4590 = call "LSPOneStatus (SubVI).vi"("VISA Refnum in"=w5015) -> ("read buffer"=w5017:string)  [unwired: 10 in]
                                n4591 = call <vilib>:"Trim Whitespace.vi"("string"=w5017) -> ("trimmed string"=w5016:string)  [unwired: 1 in]
                                n4592 = Equal?(x=w5016, y="/0`\u0003") -> (x = y?=w5014:bool)
                                n4593 = Greater Or Equal?(x=w5012, y=w5011) -> (x >= y?=w5009:bool)
                                n4594 = Or(x=w5010, y=w5009) -> (x .or. y?=w5008:bool)
                                n4595 = Or(x=w5014, y=w5008) -> (x .or. y?=w5013:bool)
                                }
                                }
                                n4596 = Wait (ms)(milliseconds to wait=u32 100) -> ()  [unwired: 1 out]
                                n4597 = local read "Stopper that ends \nthe main loops"() -> (w4978:bool)
                                n4598 = case shown="True" w4978 {
                                frame False {
                                }
                                frame True {
                                n4599 = local read "VISA Refnum in\nfor Pump"() -> (w4985:refnum<visa-resource-name>)
                                n4600 = call "HardStopCurrentProcess (SubVI).vi"("VISA Refnum in"=w4985) -> ()  [unwired: 11 in]
                                }
                                }
                                }
                              }
                              frame #7 {
                                n4601 = local write "Valve V4 Open"(TRUE ("Valve V4 Open")) -> ()
                                n4602 = local write "Valve V1 Open"(FALSE ("Valve V1 Open")) -> ()
                                n4603 = local write "Valve V2 Open"(FALSE ("Valve V2 Open")) -> ()
                                n4604 = local write "Valve V3 Open"(TRUE ("Valve V3 Open")) -> ()
                                n4605 = local write "External Valve \nOpen"(FALSE ("External Valve \nOpen")) -> ()
                                n4606 = local write "Valve V8 Open"(FALSE ("Valve V8 Open")) -> ()
                                n4607 = local write "Valve V7 Open"(TRUE ("Valve V7 Open")) -> ()
                                n4608 = local write "Valve V5 Open"(TRUE ("Valve V5 Open")) -> ()
                                n4609 = local write "Valve V6 Open"(TRUE ("Valve V6 Open")) -> ()
                              }
                              frame #8 {
                                n4610 = local read "Buffer-C1 Pumping\nResolution \nfor Equilibration \nof Column-2"() -> (w5029:T2)
